vi "Untitled 17.vi"() -> ()   [LabVIEW 2015]
panel:
  out "Array":string[](array[string])=["0.0PanelControl", "檢測項目", "4.0功能-檢測", "11.光源控制", "10.0對話視窗", "9.0功能-機台驗證", "8.0離開", "7.0等待", "6.0 錯誤", "5.0功能-檔案", "3.0功能-影像控制", "2.0功能-相機控制", "1.0 功能-IO控制"]
  in  "0.0PanelControl":T1(ring)
  in  "檢測項目":enum16{"FindPositionXY", "Match"}(ring)
  in  "4.0功能-檢測":enum16{"1.檢測-初始化", "2.浪代-浪代"}(ring)
  in  "11.0-光源控制":T2(ring)
  in  "10.0-對話視窗":enum16{""}(ring)
  in  "9.0功能-機台驗證":enum16{"1.機台驗證-初始化", "2.機台驗證-檢測"}(ring)
  in  "8.0-離開":enum16{""}(ring)
  in  "7.0-等待":enum16{"1.等待(計算時間)"}(ring)
  in  "6.0-錯誤":enum16{""}(ring)
  in  "5.0功能-檔案":T3(ring)
  in  "3.0功能-影像控制":enum16{"1.影像-初始化", "2.影像-更新影像", "3.影像-儲存影像"}(ring)
  in  "2.0功能-相機控制":enum16{"1.相機-初始化", "2.相機-取像", "3.相機-關閉"}(ring)
  in  "1.0 功能-IO控制":T4(ring)
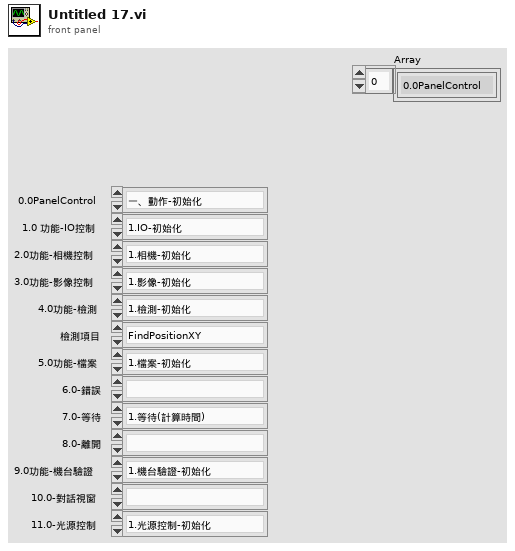
[diagram p1: front panel]
types:
  T1 = enum16{"一、動作-初始化", "二、動作-單次取像", "三、動作-連續取像", "四、動作-單步測試", "五、動作-連續測試", "六、動作-離開"}
  T2 = enum16{"1.光源控制-初始化", "2.光源控制-光源開啟", "3.光源控制-光源關閉", "4.光源控制-通訊關閉"}
  T3 = enum16{"1.檔案-初始化", "2.檔案-儲存檔案", "3.檔案-開啟檔案", "4.檔案-匯入檔案"}
  T4 = enum16{"1.IO-初始化", "2. Set Point(EOT On)", "3.Set Point(EOT Off)", "4.Get Point(SOT)"}
  T5 = cluster{"Message":string, "Message Data":variant}
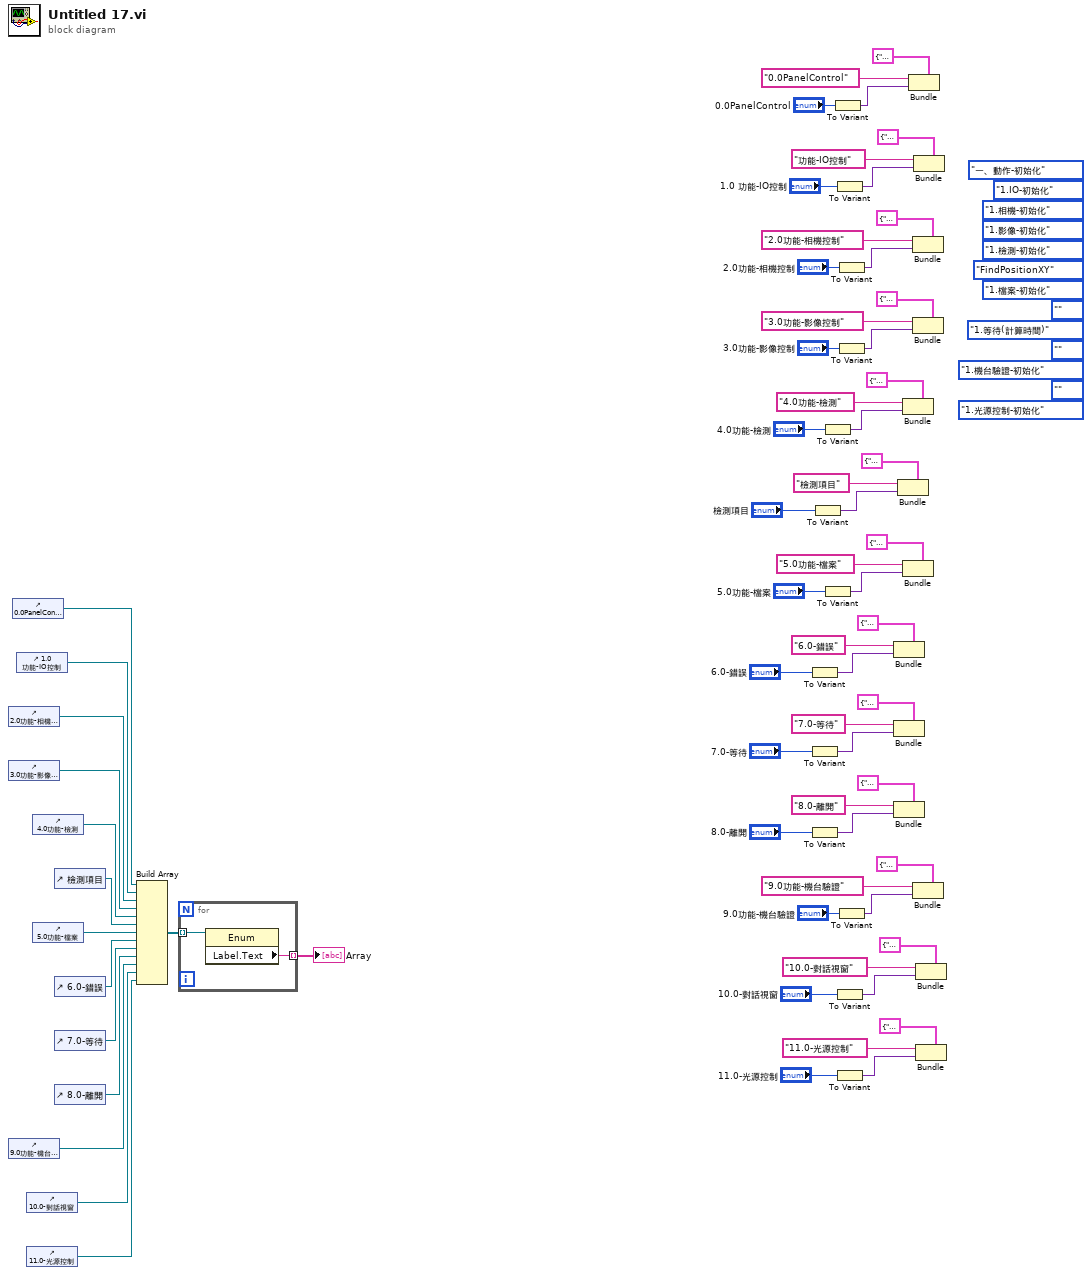
[diagram p0: block diagram]
diagram:
  (unwired) T2."1.光源控制-初始化" ("11.光源控制")
  (unwired) enum16{""}."" ("10.0對話視窗")
  (unwired) enum16{"1.機台驗證-初始化", "2.機台驗證-檢測"}."1.機台驗證-初始化" ("9.0功能-機台驗證")
  (unwired) enum16{""}."" ("8.0離開")
  (unwired) enum16{"1.等待(計算時間)"}."1.等待(計算時間)" ("7.0等待")
  (unwired) enum16{""}."" ("6.0 錯誤")
  (unwired) T3."1.檔案-初始化" ("5.0功能-檔案")
  (unwired) enum16{"FindPositionXY", "Match"}."FindPositionXY" ("檢測項目")
  (unwired) enum16{"1.檢測-初始化", "2.浪代-浪代"}."1.檢測-初始化" ("4.0功能-檢測")
  (unwired) enum16{"1.影像-初始化", "2.影像-更新影像", "3.影像-儲存影像"}."1.影像-初始化" ("3.0功能-影像控制")
  (unwired) enum16{"1.相機-初始化", "2.相機-取像", "3.相機-關閉"}."1.相機-初始化" ("2.0功能-相機控制")
  (unwired) T4."1.IO-初始化" ("1.0 功能-IO控制")
  (unwired) T1."一、動作-初始化" ("0.0PanelControl")
  n1 = control-ref of="2.0功能-相機控制"() -> (w64:refnum<vi>)
  n2 = control-ref of="3.0功能-影像控制"() -> (w63:refnum<vi>)
  n3 = control-ref of="9.0功能-機台驗證"() -> (w56:refnum<vi>)
  n4 = control-ref of="0.0PanelControl"() -> (w66:refnum<vi>)
  n5 = control-ref of="1.0 功能-IO控制"() -> (w65:refnum<vi>)
  n6 = control-ref of="10.0-對話視窗"() -> (w55:refnum<vi>)
  n7 = control-ref of="11.0-光源控制"() -> (w54:refnum<vi>)
  n8 = control-ref of="4.0功能-檢測"() -> (w62:refnum<vi>)
  n9 = control-ref of="5.0功能-檔案"() -> (w60:refnum<vi>)
  n10 = control-ref of="檢測項目"() -> (w61:refnum<vi>)
  n11 = control-ref of="6.0-錯誤"() -> (w59:refnum<vi>)
  n12 = control-ref of="7.0-等待"() -> (w58:refnum<vi>)
  n13 = control-ref of="8.0-離開"() -> (w57:refnum<vi>)
  n14 = Build Array(w66, w65, w64, w63, w62, w61, w60, w59, w58, w57, w56, w55, w54) -> (w67:refnum<vi>[])
  n15 = for {
    tunnel: w67 -> [w68] mode=indexing
    tunnel: [w69] -> w53 mode=indexing
    n16 = property class="Enum"(reference=w68) -> ("Label.Text"=w69:string)  [unwired: 1 in, 2 out]
  }
  "Array" <- w53
  n17 = To Variant(anything="6.0-錯誤") -> (Variant=w6:variant)
  n18 = To Variant(anything="7.0-等待") -> (Variant=w5:variant)
  n19 = To Variant(anything="8.0-離開") -> (Variant=w4:variant)
  n20 = To Variant(anything="檢測項目") -> (Variant=w8:variant)
  n21 = To Variant(anything="4.0功能-檢測") -> (Variant=w9:variant)
  n22 = To Variant(anything="5.0功能-檔案") -> (Variant=w7:variant)
  n23 = To Variant(anything="0.0PanelControl") -> (Variant=w37:variant)
  n24 = To Variant(anything="1.0 功能-IO控制") -> (Variant=w12:variant)
  n25 = To Variant(anything="10.0-對話視窗") -> (Variant=w2:variant)
  n26 = To Variant(anything="11.0-光源控制") -> (Variant=w1:variant)
  n27 = To Variant(anything="2.0功能-相機控制") -> (Variant=w11:variant)
  n28 = To Variant(anything="3.0功能-影像控制") -> (Variant=w10:variant)
  n29 = To Variant(anything="9.0功能-機台驗證") -> (Variant=w3:variant)
  n30 = Bundle(cluster=T5 {"Message"="", "Message Data"=variant} ("element"), "Message"="6.0-錯誤" ("Label.Text"), "Message Data"=w6) -> ()  [unwired: 1 out]
  n31 = Bundle(cluster=T5 {"Message"="", "Message Data"=variant} ("element"), "Message"="7.0-等待" ("Label.Text"), "Message Data"=w5) -> ()  [unwired: 1 out]
  n32 = Bundle(cluster=T5 {"Message"="", "Message Data"=variant} ("element"), "Message"="8.0-離開" ("Label.Text"), "Message Data"=w4) -> ()  [unwired: 1 out]
  n33 = Bundle(cluster=T5 {"Message"="", "Message Data"=variant} ("element"), "Message"="檢測項目" ("Label.Text"), "Message Data"=w8) -> ()  [unwired: 1 out]
  n34 = Bundle(cluster=T5 {"Message"="", "Message Data"=variant} ("element"), "Message"="4.0功能-檢測" ("Label.Text"), "Message Data"=w9) -> ()  [unwired: 1 out]
  n35 = Bundle(cluster=T5 {"Message"="", "Message Data"=variant} ("element"), "Message"="5.0功能-檔案" ("Label.Text"), "Message Data"=w7) -> ()  [unwired: 1 out]
  n36 = Bundle(cluster=T5 {"Message"="", "Message Data"=variant} ("element"), "Message"="0.0PanelControl" ("Label.Text"), "Message Data"=w37) -> ()  [unwired: 1 out]
  n37 = Bundle(cluster=T5 {"Message"="", "Message Data"=variant} ("element"), "Message"="2.0功能-相機控制" ("Label.Text"), "Message Data"=w11) -> ()  [unwired: 1 out]
  n38 = Bundle(cluster=T5 {"Message"="", "Message Data"=variant} ("element"), "Message"="3.0功能-影像控制" ("Label.Text"), "Message Data"=w10) -> ()  [unwired: 1 out]
  n39 = Bundle(cluster=T5 {"Message"="", "Message Data"=variant} ("element"), "Message"="9.0功能-機台驗證" ("Label.Text"), "Message Data"=w3) -> ()  [unwired: 1 out]
  n40 = Bundle(cluster=T5 {"Message"="", "Message Data"=variant} ("element"), "Message"="功能-IO控制" ("Label.Text"), "Message Data"=w12) -> ()  [unwired: 1 out]
  n41 = Bundle(cluster=T5 {"Message"="", "Message Data"=variant} ("element"), "Message"="10.0-對話視窗" ("Label.Text"), "Message Data"=w2) -> ()  [unwired: 1 out]
  n42 = Bundle(cluster=T5 {"Message"="", "Message Data"=variant} ("element"), "Message"="11.0-光源控制" ("Label.Text"), "Message Data"=w1) -> ()  [unwired: 1 out]
